vi "VI Ref FGV.vi"(7 "Check in":bool, 8 "error in (no error)":errorcluster, 10 "Ref in":refnum<vi>, 11 "Name":string) -> (0 "error out":errorcluster, 2 "Found?":bool, 3 "Ref out":refnum<vi>)   [LabVIEW 2015, in "VI.lvlib"]
uses:
  VI.lvlib
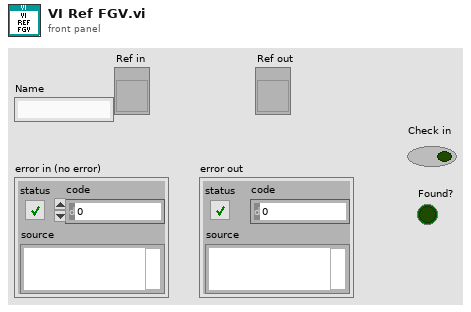
[diagram p1: front panel]
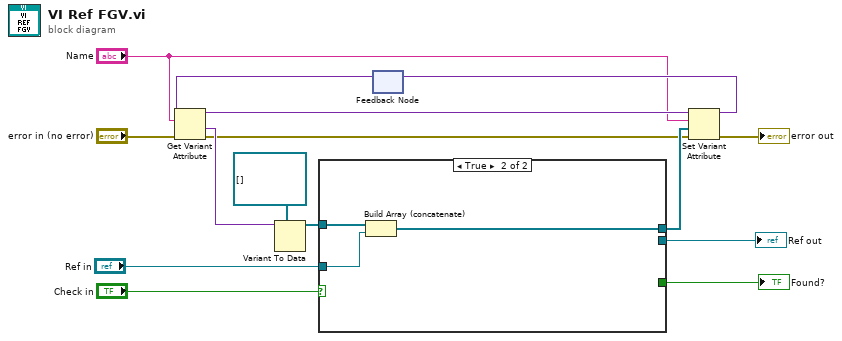
[diagram p0: block diagram]
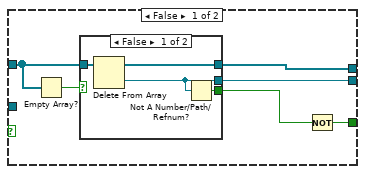
[diagram p2: hidden frame]
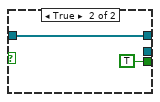
[diagram p3: hidden frame]
diagram:
  n1 = feedback #1() -> (w11:variant)  [unwired: 1 in]
  n2 = Get Variant Attribute(Variant=w11, name="Name", error in="error in (no error)") -> (duplicate Variant=w6:variant, value=w13:variant, error out=w4:errorcluster)  [unwired: 1 in, 1 out]
  n3 = Variant To Data(type=refnum<vi>[] [], Variant=w13) -> (data=w10:refnum<vi>[])  [unwired: 1 in, 1 out]
  n4 = case shown="True" "Check in" {
    tunnel: [w21 _] -> w2
    tunnel: [w20 _] -> w15
    tunnel: w10 -> [w19 w30]
    tunnel: [w18 w28] -> w7
    tunnel: "Ref in" -> [_ w29]
    frame False {
      n5 = Empty Array?(array=w19) -> (empty?=w17:bool)
      n6 = case shown="False" w17 {
        tunnel: w19 -> [w25 w27]
        tunnel: [w22 _] -> w21
        tunnel: [w24 w27] -> w18
        tunnel: [w23 TRUE] -> w16
        frame False {
          n7 = Delete From Array(array=w25) -> (deleted portion=w22:refnum<vi>, array with subset deleted=w24:refnum<vi>[])  [unwired: 2 in]
          n8 = Not A Number/Path/Refnum?(number/path/refnum=w22) -> (NaN/Path/Refnum?=w23:bool)
        }
        frame True {
        }
      }
      n9 = Not(x=w16) -> (.not. x?=w20:bool)
    }
    frame True {
      n10 = Build Array (concatenate)(w30, w29) -> (w28:refnum<vi>[])
    }
  }
  "Found?" <- w15
  "Ref out" <- w2
  n11 = Set Variant Attribute(Variant=w6, name="Name", value=w7, error in=w4) -> (Variant out=w9:variant, error out=→"error out":errorcluster)  [unwired: 1 out]
  n12 = feedback-in #1(w9) -> ()
